vi "OpenH5WithAttr.vi"(5 "Filename":string, 6 "Additional Info":T1, 7 "File Directory":path, 8 "error in (no error)":errorcluster, 9 "Generator Info":T3, 10 "Digitizer Info":T5, 11 "Stage Setup Info":T6) -> (0 "error out":errorcluster, 3 "HDF5 Ref out":T2)   [LabVIEW 2018]
uses:
  D:/HardwareRevamp/AcustoXv2/Controls/StageInfo.ctl
  D:/HardwareRevamp/AcustoXv2/Controls/DigitizerInfo.ctl
  <vilib>/userdefined/High Color/nirio_resource_hc.ctl
  D:/HardwareRevamp/AcustoXv2/Controls/GeneratorInfo.ctl
  <vilib>/UPVI/lvhdf5/library.llb/HDF5 Ref.ctl
  D:/HardwareRevamp/AcustoXv2/Controls/AdditionalData.ctl
  <vilib>/UPVI/lvhdf5/file.llb/LVH5F Operation.ctl
  <vilib>/UPVI/lvhdf5/group.llb/OpenCreateGroup (String).vi
  <vilib>/UPVI/lvhdf5/attribute.llb/Write Multiple Attributes.vi
  <vilib>/UPVI/lvhdf5/attribute.llb/LVH5A Operation.ctl
  <vilib>/UPVI/lvhdf5/attribute.llb/LVH5 Write Attributes.xnode
  <vilib>/Utility/VariantDataType/GetClusterInfo.vi
  <vilib>/Utility/VariantDataType/VariantType.lvlib
  <vilib>/Utility/VariantDataType/GetTypeInfo.vi
  <vilib>/UPVI/lvhdf5/attribute.llb/Cluster to Attribute Array.xnode
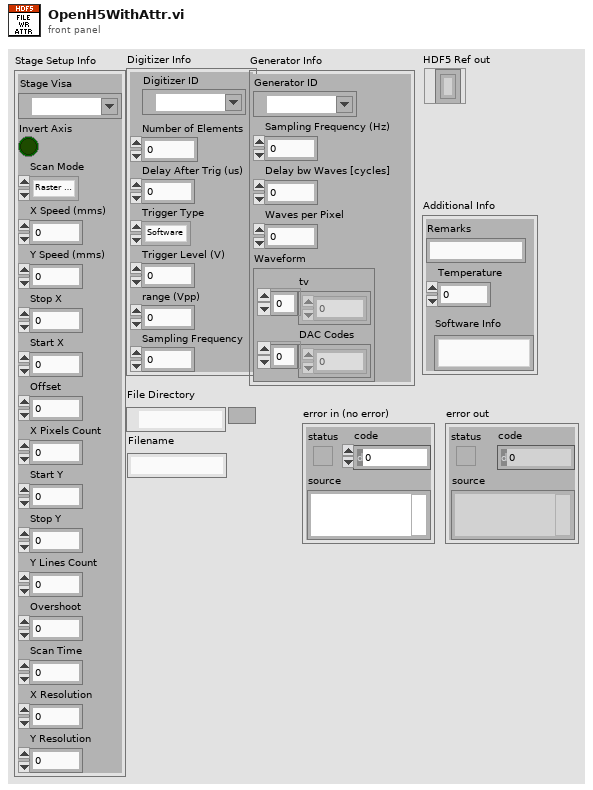
[diagram p1: front panel]
types:
  T1 = typedef "AdditionalData.ctl" = cluster{"Remarks":string, "Temperature":dbl, "Software Info":string}
  T2 = typedef "HDF5 Ref.ctl" = refnum<k1>
  T3 = typedef "GeneratorInfo.ctl" = cluster{"Generator ID":T4, "Sampling Frequency (Hz)":u64, "Delay bw Waves [cycles]":u16, "Waves per Pixel":u32, "Waveform":cluster{"tv":dbl[], "DAC Codes":u16[]}}
  T4 = typedef "nirio_resource_hc.ctl" = tag
  T5 = typedef "DigitizerInfo.ctl" = cluster{"Digitizer ID":T4, "Number of Elements":u16, "Delay After Trig (us)":dbl, "Trigger Type":enum8{"Software", "Data Edge"}, "Trigger Level (V)":dbl, "range (Vpp)":dbl, "Sampling Frequency":dbl}
  T6 = typedef "StageInfo.ctl" = cluster{"Stage Visa":refnum<visa-resource-name>, "Invert Axis":bool, "Scan Mode":enum16{"Raster Scan", "Serpentine Scan"}, "X Speed (mms)":dbl, "Y Speed (mms)":dbl, "Stop X":dbl, "Start X":dbl, "Offset":dbl, "X Pixels Count":i32, "Start Y":dbl, "Stop Y":dbl, "Y Lines Count":i32, "Overshoot":dbl, "Scan Time":dbl, "X Resolution":dbl, "Y Resolution":dbl}
  T7 = typedef "LVH5F Operation.ctl" = enum16{"open", "open or create", "create or replace", "create or replace (with confirmation)", "create", "open (read only)"}
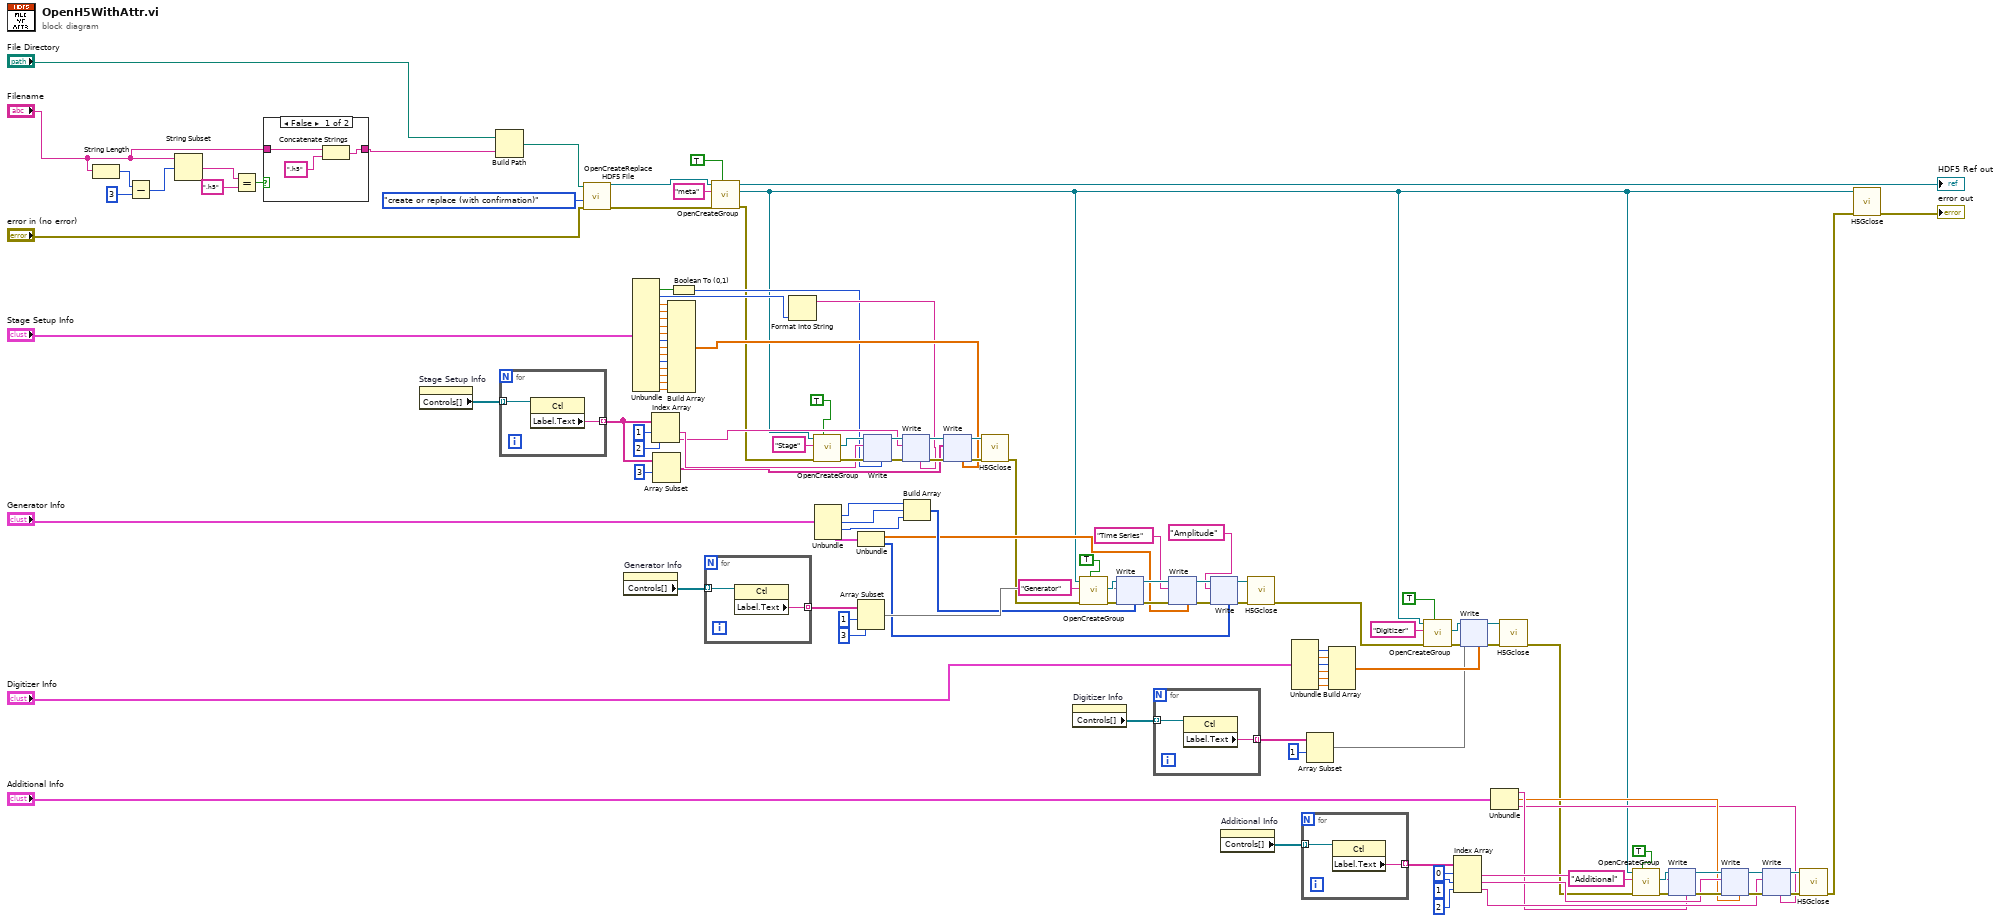
[diagram p0: block diagram]
diagram:
  n1 = String Length(string="Filename") -> (length=w34:i32)
  n2 = Subtract(x=w34, y=3) -> (x-y=w33:i32)
  n3 = String Subset(string="Filename", offset (0)=w33) -> (substring=w31:string)  [unwired: 1 in]
  n4 = Equal?(x=w31, y=".h5") -> (x = y?=w29:bool)
  n5 = case shown="False" w29 {
    tunnel: "Filename" -> [w129 w130]
    tunnel: [w128 w130] -> w28
    frame False {
      n6 = Concatenate Strings(w129, ".h5" ("y")) -> (w128:string)
    }
    frame True {
    }
  }
  n7 = property on="Stage Setup Info" class="Clust (strict)"() -> ("Controls[]"=w126:refnum<vi>[])  [unwired: 2 in, 2 out]
  n8 = Build Path(base path="File Directory", name or relative path=w28) -> (appended path=w36:path)
  n9 = for {
    tunnel: w126 -> [w132] mode=indexing
    tunnel: [w131] -> w86 mode=indexing
    n10 = property on="Property Node" class="Ctl"(reference=w132) -> ("Label.Text"=w131:string)  [unwired: 1 in, 2 out]
  }
  n11 = call <vilib>:"OpenCreateReplace HDF5 File.vi"("error in (no error)"="error in (no error)", "function (open or create)"=LVH5F_Operation."create or replace (with confirmation)", "path"=w36) -> ("error out"=w40:errorcluster, "HDF5 Ref out"=w39:T2)  [unwired: 5 in]
  n12 = property on="Generator Info" class="Clust (strict)"() -> ("Controls[]"=w73:refnum<vi>[])  [unwired: 2 in, 2 out]
  n13 = Unbundle("Stage Setup Info") -> ("Invert Axis"=w77:bool, "Scan Mode"=w79:enum16{"Raster Scan", "Serpentine Scan"}, "X Speed (mms)"=w124:dbl, "Y Speed (mms)"=w123:dbl, "Stop X"=w122:dbl, "Start X"=w121:dbl, "Offset"=w120:dbl, "X Pixels Count"=w119:i32, "Start Y"=w118:dbl, "Stop Y"=w117:dbl, "Y Lines Count"=w116:i32, "Overshoot"=w115:dbl, "Scan Time"=w114:dbl, "X Resolution"=w113:dbl, "Y Resolution"=w112:dbl)  [unwired: 1 out]
  n14 = Index Array(array=w86, index #1=1 ("index"), index #2=2 ("index")) -> (element #1=w84:string, element #2=w83:string)
  n15 = Array Subset(array=w86, index=3) -> (w82:string[])  [unwired: 1 in]
  n16 = Build Array(w124, w123, w122, w121, w120, w119, w118, w117, w116, w115, w114, w113, w112) -> (w81:dbl[])
  n17 = Boolean To (0,1)(Boolean=w77) -> (0, 1=w76:i16)
  n18 = for {
    tunnel: w73 -> [w134] mode=indexing
    tunnel: [w133] -> w74 mode=indexing
    n19 = property on="Property Node" class="Ctl"(reference=w134) -> ("Label.Text"=w133:string)  [unwired: 1 in, 2 out]
  }
  n20 = call-poly <vilib>:"OpenCreateGroup.vi"("Create if not found (F)"=TRUE, "error in (no error)"=w40, "Group"="meta", "HDF5 Ref"=w39) -> ("error out"=w43:errorcluster, "HDF5 Group Ref"=w1:T2, "HDF5 Ref out"=→"HDF5 Ref out":T2)  [unwired: 5 in]
  n21 = Format Into String(w79) -> (resulting string=w78:string)  [unwired: 3 in, 1 out]
  n22 = call-poly <vilib>:"OpenCreateGroup.vi"("Create if not found (F)"=TRUE, "error in (no error)"=w43, "Group"="Stage", "HDF5 Ref"=w1) -> ("error out"=w107:errorcluster, "HDF5 Group Ref"=w104:T2)  [unwired: 5 in, 1 out]
  n23 = Unbundle("Generator Info") -> ("Sampling Frequency (Hz)"=w70:u64, "Delay bw Waves [cycles]"=w69:u16, "Waves per Pixel"=w68:u32, "Waveform"=w71:cluster{"tv":dbl[], "DAC Codes":u16[]})  [unwired: 1 out]
  n24 = Unbundle(w71) -> ("tv"=w62:dbl[], "DAC Codes"=w61:u16[])
  n25 = Array Subset(array=w74, index=1, length=3) -> (w66:string[])
  n26 = xnode "Write"("HDF5 Ref"=w104, "error in (no error)"=w107, "Name(s)"=w84, "Value(s)"=w76) -> ("HDF5 Ref out"=w111:T2, "error out"=w110:errorcluster)  [unwired: 1 in]
  n27 = xnode "Write"("HDF5 Ref"=w111, "error in (no error)"=w110, "Name(s)"=w83, "Value(s)"=w78) -> ("HDF5 Ref out"=w109:T2, "error out"=w108:errorcluster)  [unwired: 1 in]
  n28 = Build Array(w70, w69, w68) -> (w65:u64[])
  n29 = xnode "Write"("HDF5 Ref"=w109, "error in (no error)"=w108, "Name(s)"=w82, "Value(s)"=w81) -> ("HDF5 Ref out"=w106:T2, "error out"=w105:errorcluster)  [unwired: 1 in]
  n30 = call <vilib>:"H5Gclose.vi"("error in (no error)"=w105, "HDF5 Group Ref"=w106) -> ("error out"=w47:errorcluster)  [unwired: 7 in]
  n31 = property on="Digitizer Info" class="Clust (strict)"() -> ("Controls[]"=w60:refnum<vi>[])  [unwired: 2 in, 2 out]
  n32 = call-poly <vilib>:"OpenCreateGroup.vi"("Create if not found (F)"=TRUE, "error in (no error)"=w47, "Group"="Generator", "HDF5 Ref"=w1) -> ("error out"=w98:errorcluster, "HDF5 Group Ref"=w101:T2)  [unwired: 5 in, 1 out]
  n33 = xnode "Write"("HDF5 Ref"=w101, "error in (no error)"=w98, "Name(s)"=w66, "Value(s)"=w65) -> ("HDF5 Ref out"=w94:T2, "error out"=w95:errorcluster)  [unwired: 1 in]
  n34 = for {
    tunnel: w60 -> [w136] mode=indexing
    tunnel: [w135] -> w59 mode=indexing
    n35 = property on="Property Node" class="Ctl"(reference=w136) -> ("Label.Text"=w135:string)  [unwired: 1 in, 2 out]
  }
  n36 = xnode "Write"("HDF5 Ref"=w94, "error in (no error)"=w95, "Name(s)"="Time Series" ("Group"), "Value(s)"=w62) -> ("HDF5 Ref out"=w96:T2, "error out"=w97:errorcluster)  [unwired: 1 in]
  n37 = xnode "Write"("HDF5 Ref"=w96, "error in (no error)"=w97, "Name(s)"="Amplitude" ("Group"), "Value(s)"=w61) -> ("HDF5 Ref out"=w99:T2, "error out"=w100:errorcluster)  [unwired: 1 in]
  n38 = property on="Additional Info" class="Clust (strict)"() -> ("Controls[]"=w25:refnum<vi>[])  [unwired: 2 in, 2 out]
  n39 = call <vilib>:"H5Gclose.vi"("error in (no error)"=w100, "HDF5 Group Ref"=w99) -> ("error out"=w48:errorcluster)  [unwired: 7 in]
  n40 = Unbundle("Digitizer Info") -> ("Number of Elements"=w56:u16, "Delay After Trig (us)"=w55:dbl, "Trigger Type"=w54:enum8{"Software", "Data Edge"}, "Trigger Level (V)"=w53:dbl, "range (Vpp)"=w52:dbl, "Sampling Frequency"=w51:dbl)  [unwired: 1 out]
  n41 = for {
    tunnel: w25 -> [w138] mode=indexing
    tunnel: [w137] -> w13 mode=indexing
    n42 = property on="Property Node" class="Ctl"(reference=w138) -> ("Label.Text"=w137:string)  [unwired: 1 in, 2 out]
  }
  n43 = Array Subset(array=w59, index=1) -> (w49:string[])  [unwired: 1 in]
  n44 = Build Array(w56, w55, w54, w53, w52, w51) -> (w50:dbl[])
  n45 = call-poly <vilib>:"OpenCreateGroup.vi"("Create if not found (F)"=TRUE, "error in (no error)"=w48, "Group"="Digitizer", "HDF5 Ref"=w1) -> ("error out"=w91:errorcluster, "HDF5 Group Ref"=w90:T2)  [unwired: 5 in, 1 out]
  n46 = Index Array(array=w13, index #1=0 ("index"), index #2=1 ("index"), index #3=2 ("index")) -> (element #1=w11:string, element #2=w10:string, element #3=w7:string)
  n47 = xnode "Write"("HDF5 Ref"=w90, "error in (no error)"=w91, "Name(s)"=w49, "Value(s)"=w50) -> ("HDF5 Ref out"=w93:T2, "error out"=w92:errorcluster)  [unwired: 1 in]
  n48 = Unbundle("Additional Info") -> ("Remarks"=w6:string, "Temperature"=w5:dbl, "Software Info"=w4:string)
  n49 = call <vilib>:"H5Gclose.vi"("error in (no error)"=w92, "HDF5 Group Ref"=w93) -> ("error out"=w2:errorcluster)  [unwired: 7 in]
  n50 = call-poly <vilib>:"OpenCreateGroup.vi"("Create if not found (F)"=TRUE, "error in (no error)"=w2, "Group"="Additional", "HDF5 Ref"=w1) -> ("error out"=w18:errorcluster, "HDF5 Group Ref"=w15:T2)  [unwired: 5 in, 1 out]
  n51 = xnode "Write"("HDF5 Ref"=w15, "error in (no error)"=w18, "Name(s)"=w11, "Value(s)"=w6) -> ("HDF5 Ref out"=w22:T2, "error out"=w21:errorcluster)  [unwired: 1 in]
  n52 = xnode "Write"("HDF5 Ref"=w22, "error in (no error)"=w21, "Name(s)"=w10, "Value(s)"=w5) -> ("HDF5 Ref out"=w20:T2, "error out"=w19:errorcluster)  [unwired: 1 in]
  n53 = xnode "Write"("HDF5 Ref"=w20, "error in (no error)"=w19, "Name(s)"=w7, "Value(s)"=w4) -> ("HDF5 Ref out"=w17:T2, "error out"=w16:errorcluster)  [unwired: 1 in]
  n54 = call <vilib>:"H5Gclose.vi"("error in (no error)"=w16, "HDF5 Group Ref"=w17) -> ("error out"=w3:errorcluster)  [unwired: 7 in]
  n55 = call <vilib>:"H5Gclose.vi"("error in (no error)"=w3, "HDF5 Group Ref"=w1) -> ("error out"=→"error out":errorcluster)  [unwired: 7 in]
